vi "Initialize Plugin.vi"(6 "Resource (blank for prompt)":string, 7 "Instance Name (blank for default)":string, 8 "error in (no error)":errorcluster, 9 "Log Directory":path, 10 "Plugin Path in":path, 11 "Plugin Type":T1) -> (0 "error out":errorcluster, 2 "Failed?":bool, 3 "Generic Controller out":refnum<class "Generic Plugin.lvclass">)   [LabVIEW 2020, in "RxnRover.lvlib"]
doc: "Initialize a plugin instance based on the information given."
uses:
  RxnRover.lvlib
  Controller/Generic Plugin.lvclass
  Controller/Controller Type.ctl
  <userlib>/RxnRover/DynamicReentrant/Dynamic Reentrant.lvlib
  logging/logging.lvlib
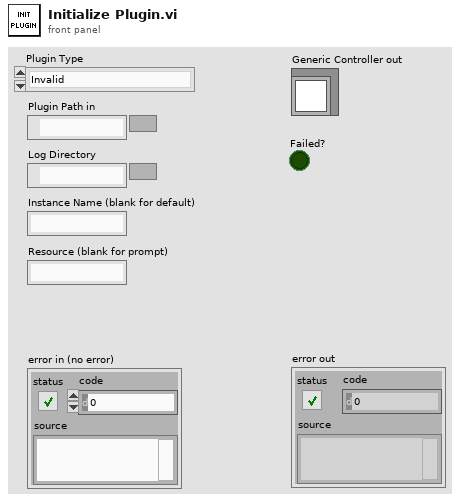
[diagram p1: front panel]
types:
  T1 = typedef "RxnRover.lvlib/Generic Plugin.lvclass/Controller Type.ctl" = enum16{"Invalid", "Temperature Controller", "Pump Controller", "Syringe Pump", "Generic Optimizer", "LC Parser", "Passive Hardware"}
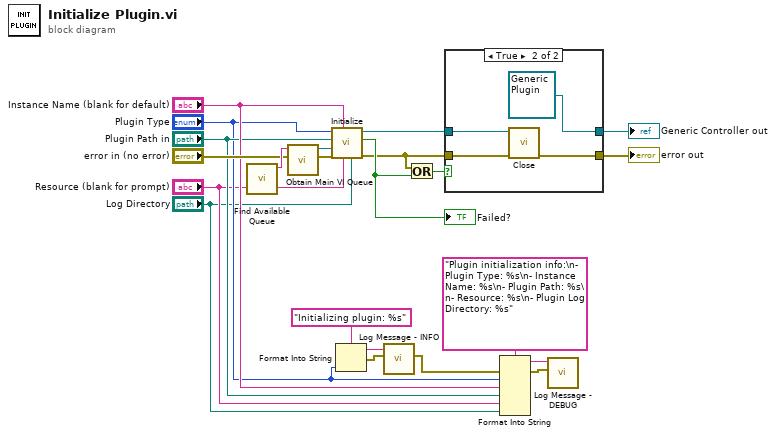
[diagram p0: block diagram]
diagram:
  n1 = call "Find Available Queue.vi"() -> ("String"=w20:string)  [unwired: 11 in]
  n2 = call <userlib>:"Obtain Main VI Queue.vi"("error in (no error)"="error in (no error)", "Name (Main VI)"=w20) -> ("error out"=w22:errorcluster, "Main VI Queue"=w21:refnum<queue>)  [unwired: 8 in]
  n3 = call "Initialize.vi"("Log Directory"="Log Directory", "Resource"="Resource (blank for prompt)", "Instance Name"="Instance Name (blank for default)", "error in (no error)"=w22, "Receiving Queue"=w21, "Control Panel Path"="Plugin Path in", "Controller Type"="Plugin Type") -> ("error out"=w16:errorcluster, "Failed?"=w17:bool, "Plugin Server out"=w14:refnum<class "Generic Plugin.lvclass">)  [unwired: 2 in]
  "Failed?" <- w17
  n4 = Format Into String(format string="Initializing plugin: %s", "Plugin Type") -> (resulting string=w8:string, error out=w7:errorcluster)  [unwired: 2 in]
  n5 = call "Log Message - INFO.vi"("error in (no error)"=w7, "Message"=w8) -> ("error out"=w6:errorcluster)  [unwired: 9 in]
  n6 = Or(x=w16, y=w17) -> (x .or. y?=w18:bool)
  n7 = case shown="True" w18 {
    tunnel: w16 -> [w23 w27]
    tunnel: [w23 w26] -> w15
    tunnel: w14 -> [w24 w28]
    tunnel: [w24 refnum<class "Generic Plugin.lvclass"> refnum ("Plugin Server out")] -> w13
    frame False {
    }
    frame True {
      n8 = call "Close.vi"("error in (no error)"=w27, "Plugin in"=w28) -> ("error out"=w26:errorcluster)  [unwired: 9 in]
    }
  }
  "error out" <- w15
  "Generic Controller out" <- w13
  n9 = Format Into String(format string="Plugin initialization info:\n- Plugin Type: %s\n- Instance Name: %s\n- Plugin Path: %s\n- Resource: %s\n- Plugin Log Directory: %s", error in=w6, "Plugin Type", "Instance Name (blank for default)", "Plugin Path in", "Resource (blank for prompt)", "Log Directory") -> (resulting string=w10:string, error out=w11:errorcluster)  [unwired: 1 in]
  n10 = call "Log Message - DEBUG.vi"("error in (no error)"=w11, "Message"=w10) -> ()  [unwired: 9 in, 1 out]
